vi "MaxZ_2019.04.08.vi"(8 "dwell_time_ms":dbl=100.0, 9 "q_steps":i32=100, 10 "z_end_um":dbl=100.0, 11 "z_start_um":dbl) -> (2 "focus_data":cluster{"Ramp Pattern":dbl[], dbl[]}(graph), 3 "z_focus_um":dbl)   [LabVIEW 2014]
uses:
  <vilib>/Analysis/1siggen.llb/Ramp Pattern by Samples.vi
  <vilib>/Analysis/NI_AALBase.lvlib
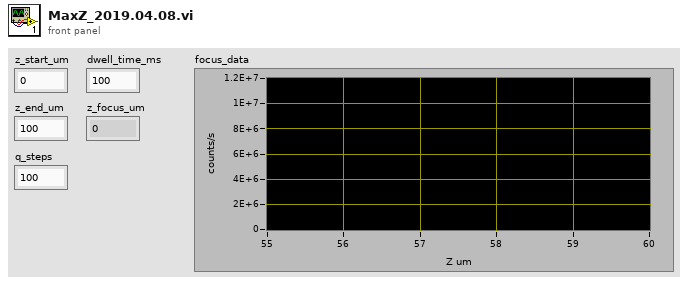
[diagram p1: front panel]
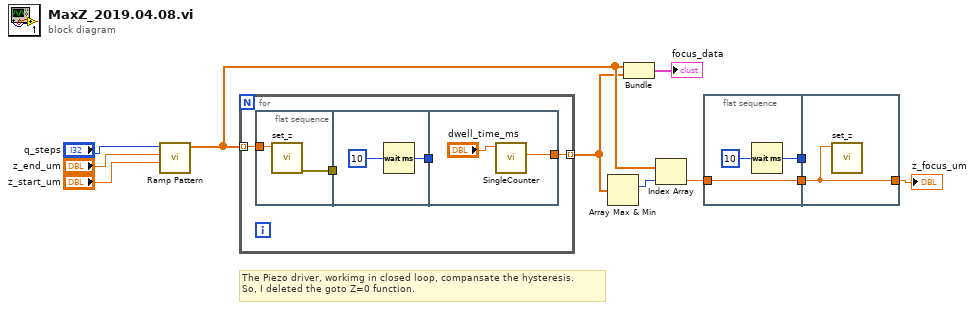
[diagram p0: block diagram]
diagram:
  # "The Piezo driver, workimg in closed loop, compansate the hysteresis.\nSo, I deleted the goto Z=0 function."
  n1 = call-poly <vilib>:"Ramp Pattern.vi"("start"="z_start_um", "end"="z_end_um", "samples"="q_steps") -> ("Ramp Pattern"=w4:dbl[])  [unwired: 7 in, 1 out]
  n2 = for {
    tunnel: w4 -> [w15] mode=indexing
    tunnel: [w14] -> w2 mode=indexing
    n3 = flat-sequence {
      tunnel: w15 -> [w17]
      tunnel: [w16] -> w13
      tunnel: w13 -> [_]
      tunnel: [w18] -> w12
      tunnel: [w20] -> w14
      tunnel: w12 -> [_]
      frame #0 {
        n4 = call "set_z.vi"("z_value_um"=w17) -> ("error out"=w16:errorcluster)  [unwired: 10 in]
      }
      frame #1 {
        n5 = Wait (ms)(milliseconds to wait=u32 10) -> (millisecond timer value=w18:u32)
      }
      frame #2 {
        n6 = call "SingleCounter.vi"("Dwell_time_ms"="dwell_time_ms") -> ("counts/s"=w20:dbl)  [unwired: 8 in, 2 out]
      }
    }
  }
  n7 = Array Max & Min(array=w2) -> (max index (indices)=w9:i32)  [unwired: 3 out]
  n8 = Bundle("Ramp Pattern"=w4, w2) -> (→"focus_data":cluster{"Ramp Pattern":dbl[], dbl[]})  [unwired: 1 in]
  n9 = Index Array(array=w4, index=w9) -> (element=w6:dbl)
  n10 = flat-sequence {
    tunnel: [w23] -> w7
    tunnel: [w22] -> w1
    tunnel: w6 -> [w23]
    tunnel: w7 -> [w25]
    tunnel: [w25] -> w5
    tunnel: w1 -> [_]
    frame #0 {
      n11 = Wait (ms)(milliseconds to wait=u32 10) -> (millisecond timer value=w22:u32)
    }
    frame #1 {
      n12 = call "set_z.vi"("z_value_um"=w25) -> ()  [unwired: 10 in, 1 out]
    }
  }
  "z_focus_um" <- w5
